vi "Write Result.vi"(0 "Scalar Charact Result Accessor in":refnum<class "Scalar Charact Result Accessor.lvclass">, 5 "Charact Result":variant, 11 "error in":errorcluster) -> (4 "Scalar Charact Result Accessor out":refnum<class "Scalar Charact Result Accessor.lvclass">, 15 "error out":errorcluster)   [LabVIEW 2023, in "RFFixtureCharact.RFPM.lvlib" / "Scalar Charact Result Accessor.lvclass"]
uses:
  Scalar Charact Result Accessor.lvclass
  C:/srd-semi-rfcal-software/AuxTools/STSRFFixtureCharactUtility/Source/Code Modules/Fixture/RFPM/Charact Result Accessor/Base/Charact Result Accessor.lvclass
  Dependencies/HFNetworkAnalysis/Controls/SnPDataType.ctl
  Public/Base Classes/Scalar/Scalar Path/Type Definitions/Scalar Charact Result.ctl
  Dependencies/HFNetworkAnalysis/NI_HFNetworkAnalysis.lvlib
  Public/Base Classes/Scalar/Scalar Path/Scalar Path.lvclass
  Base/Charact Result Accessor.lvclass
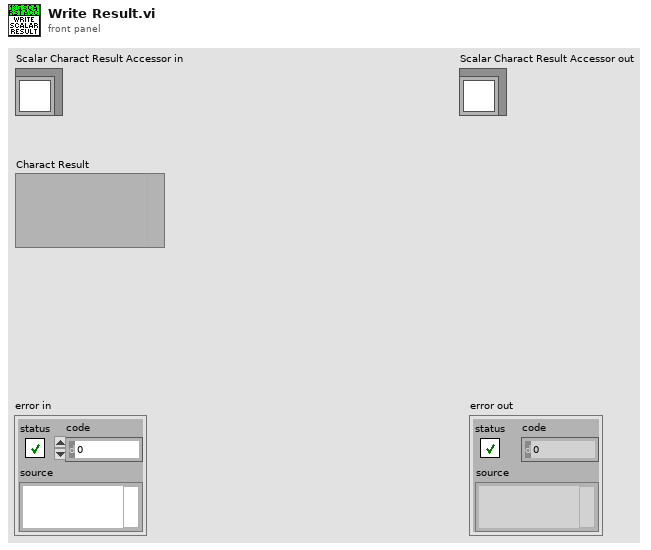
[diagram p1: front panel]
types:
  T1 = typedef "RFFixtureCharact.Public.lvlib/Scalar Path.lvclass/Scalar Charact Result.ctl" = cluster{"Port Power":dbl, "Reference Level":dbl, "Frequency":dbl, "Path Gain":dbl, "Out Of Limit":bool}
  T2 = typedef "NI_HFNetworkAnalysis.lvlib/SnPDataType.ctl" = enum16{"DB", "MA", "RI"}
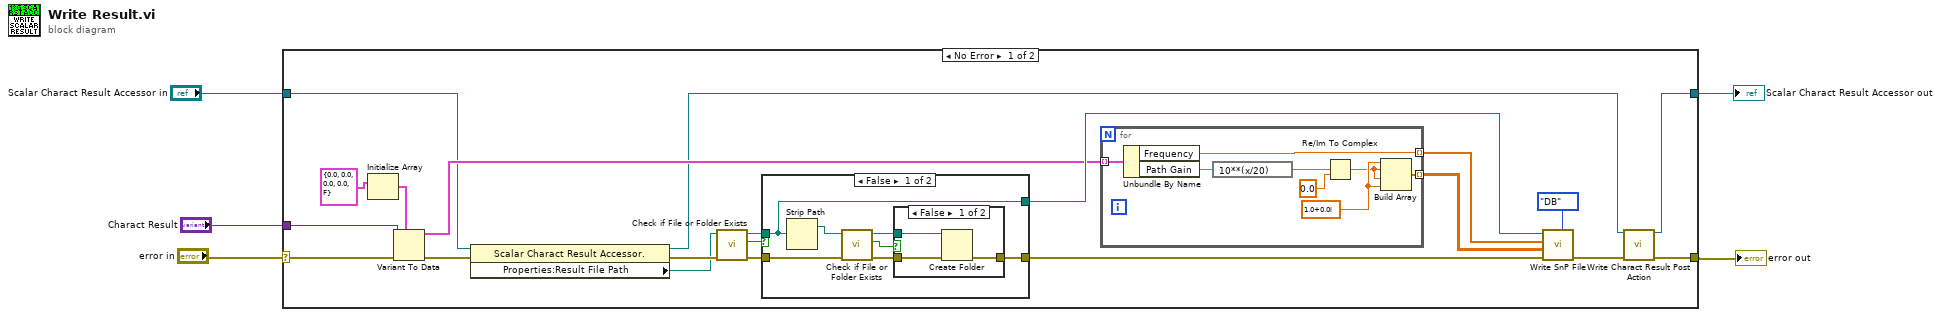
[diagram p0: block diagram]
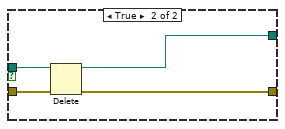
[diagram p3: hidden frame]
diagram:
  n1 = case shown="No Error" "error in" {
    selector: "error in" -> [w16 w51]
    tunnel: [w8 w51] -> w1
    tunnel: "Charact Result" -> [w15 _]
    tunnel: "Scalar Charact Result Accessor in" -> [w11 w50]
    tunnel: [w6 w50] -> w2
    frame No Error {
      n2 = Initialize Array(T1 {"Port Power"=0.0, "Reference Level"=0.0, "Frequency"=0.0, "Path Gain"=0.0, "Out Of Limit"=FALSE} ("Charact Result")) -> (w17:T1[])  [unwired: 1 in]
      n3 = Variant To Data(error in=w16, type=w17, Variant=w15) -> (data=w14:T1[], error out=w13:errorcluster)
      n4 = property class="Scalar Charact Result Accessor."(reference=w11, error in=w13) -> (reference out=w7:refnum<class "Scalar Charact Result Accessor.lvclass">, error out=w12:errorcluster, "Properties:Result File Path"=w10:path)
      n5 = call <vilib>:"Check if File or Folder Exists.vi"("error in (no error)"=w12, "path"=w10) -> ("error out"=w22:errorcluster, "file or folder exists?"=w21:bool, "dup path"=w20:path)  [unwired: 7 in]
      n6 = case shown="False" w21 {
        tunnel: [w28 w41] -> w19
        tunnel: [w27 w40] -> w23
        tunnel: w22 -> [w30 w39]
        tunnel: w20 -> [w27 w38]
        frame False {
          n7 = Strip Path(path=w27) -> (stripped path=w29:path)  [unwired: 1 out]
          n8 = call <vilib>:"Check if File or Folder Exists.vi"("error in (no error)"=w30, "path"=w29) -> ("error out"=w31:errorcluster, "file or folder exists?"=w33:bool, "dup path"=w32:path)  [unwired: 7 in]
          n9 = case shown="False" w33 {
            tunnel: w31 -> [w36 w37]
            tunnel: [w35 w37] -> w28
            tunnel: w32 -> [w34 _]
            frame False {
              n10 = Create Folder(path (use dialog)=w34, error in=w36) -> (error out=w35:errorcluster)  [unwired: 1 in, 2 out]
            }
            frame True {
            }
          }
        }
        frame True {
          n11 = Delete(path (use dialog)=w38, error in=w39) -> (deleted path=w40:path, error out=w41:errorcluster)  [unwired: 3 in, 1 out]
        }
      }
      n12 = for {
        tunnel: w14 -> [w49] mode=indexing
        tunnel: [w48] -> w26 mode=indexing
        tunnel: [w47] -> w25 mode=indexing
        w45 = cdb 1.0+0.0i ("element")
        n13 = Unbundle By Name(w49) -> ("Frequency"=w48:dbl, "Path Gain"=w44:dbl)
        n14 = expression code="10**(x/20)"(w44) -> (w43:dbl)
        n15 = Re/Im To Complex(1:0.0 ("y"), 2:w43) -> (0:w42:cdb)
        n16 = Build Array(w45, w42, w42, w45) -> (w47:cdb[])
      }
      n17 = call "Write SnP File.vi"("OutputDataType"=SnPDataType."DB", "error in (no error)"=w19, "S-parameters"=w25, "Frequencies (Hz)"=w26, "SnP File Path"=w23) -> ("error out"=w9:errorcluster)  [unwired: 6 in]
      n18 = call "Write Charact Result Post Action.vi"("Charact Result Accessor in"=w7, "error in"=w9) -> ("Charact Result Accessor out"=w6:refnum<class "Scalar Charact Result Accessor.lvclass">, "error out"=w8:errorcluster)  [unwired: 12 in]
    }
    frame Error {
    }
  }
  "error out" <- w1
  "Scalar Charact Result Accessor out" <- w2
